vi "Extract Strings from Menu.vi"(8 "error in (no error)":errorcluster, 11 "Object in":refnum<class "Menu Data.lvclass">) -> (0 "error out":errorcluster, 3 "Object out":refnum<class "Menu Data.lvclass">)   [LabVIEW 2013, in "SET Project Data.lvlib" / "Menu Data.lvclass"]
uses:
  Menu Data.lvclass
  Menu Data.lvclass/Menu Data.ctl
  <vilib>/Utility/miscctls.llb/LVMenuShortCut.ctl
  Resource Data Class/Resource Data.lvclass
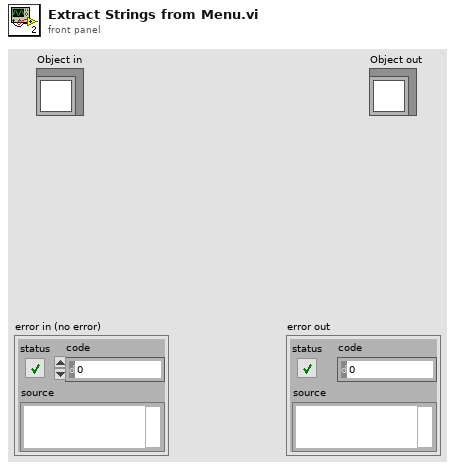
[diagram p1: front panel]
types:
  T1 = enum32{"Invalid", "Standard", "Closed", "Hidden", "Minimized", "Maximized"}
  T2 = typedef "LVMenuShortCut.ctl" = cluster{"Include Shift Key?":bool, "Include Ctrl Key?":bool, "Shortcut Key":string}
  T3 = cluster{"tag":string, "name":string, "short cut":T2, "enabled":bool, "checked":bool}[]
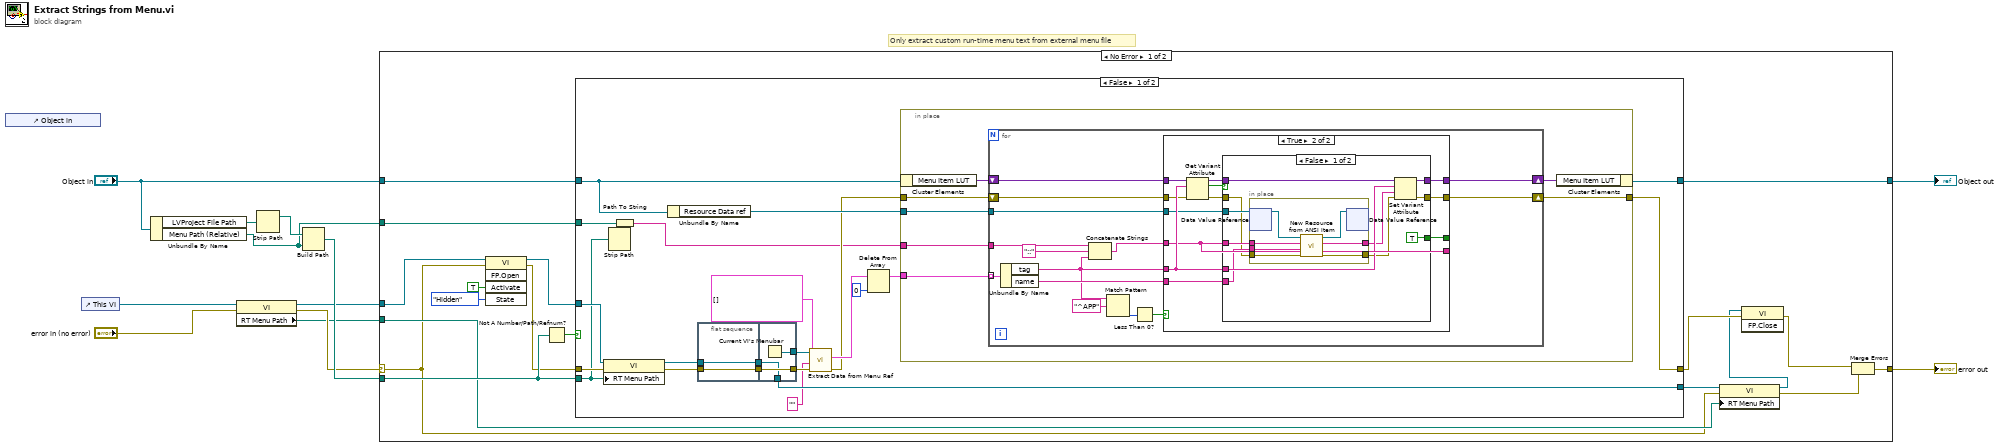
[diagram p0: block diagram]
diagram:
  # "Only extract custom run-time menu text from external menu file"
  n1 = control-ref of="Object in"() -> ()  [unwired: 1 out]
  n2 = control-ref of="This VI"() -> (w6:refnum<vi>)
  n3 = Unbundle By Name("Object in") -> ("LVProject File Path"=w11:path, "Menu Path (Relative)"=w1:path)
  n4 = property class="VI"(reference=w6, error in="error in (no error)") -> (reference out=w5:refnum<vi>, error out=w3:errorcluster, "RT Menu Path"=w2:path)
  n5 = Strip Path(path=w11) -> (stripped path=w12:path)  [unwired: 1 out]
  n6 = Build Path(base path=w12, name or relative path=w1) -> (appended path=w8:path)
  n7 = case shown="No Error" w3 {
    selector: w3 -> [w19 w118]
    tunnel: w5 -> [w23 _]
    tunnel: [w26 w118] -> w7
    tunnel: w8 -> [w29 _]
    tunnel: "Object in" -> [w28 w117]
    tunnel: [w27 w117] -> w9
    tunnel: w2 -> [w24 _]
    tunnel: w1 -> [w13 _]
    frame No Error {
      n8 = invoke class="VI" method="FP.Open"(reference=w23, error in=w19, "Activate"=TRUE ("Activate?"), "State"=T1."Hidden") -> (reference out=w22:refnum<vi>, error out=w18:errorcluster)  [unwired: 1 in, 3 out]
      n9 = Not A Number/Path/Refnum?(number/path/refnum=w29) -> (NaN/Path/Refnum?=w30:bool)
      n10 = case shown="False" w30 {
        tunnel: w22 -> [w51 w114]
        tunnel: w18 -> [w50 w116]
        tunnel: [w40 w116] -> w16
        tunnel: w29 -> [w44 _]
        tunnel: w28 -> [w43 w115]
        tunnel: [w45 w115] -> w27
        tunnel: [w36 w114] -> w17
        tunnel: w13 -> [w32 _]
        frame False {
          n11 = property class="VI"(reference=w51, error in=w50, "RT Menu Path"=w44) -> (reference out=w37:refnum<vi>, error out=w39:errorcluster)
          n12 = Strip Path(path=w44) -> ()  [unwired: 2 out]
          n13 = Path To String(path=w32) -> (string=w31:string)
          n14 = Unbundle By Name(w43) -> ("Resource Data ref"=w42:refnum<data-value>)
          n15 = flat-sequence {
            tunnel: w39 -> [w110]
            tunnel: [w110] -> w38
            tunnel: w37 -> [w109]
            tunnel: [w109] -> w35
            tunnel: [w113] -> w52
            tunnel: [w112] -> w49
            tunnel: w38 -> [w112]
            tunnel: [w111] -> w36
            tunnel: w35 -> [w111]
            frame #0 {
            }
            frame #1 {
              n16 = Current VI's Menubar() -> (w113:refnum<k9>)
            }
          }
          n17 = call "Extract Data from Menu Ref.vi"("error in (no error)"=w49, "Starting Tag"="", "Menu Items in"=T3 [], "menu reference"=w52) -> ("error out"=w41:errorcluster, "Menu Items out"=w48:T3)  [unwired: 5 in, 1 out]
          n18 = Delete From Array(array=w48, index=0) -> (array with subset deleted=w47:T3)  [unwired: 1 in, 1 out]
          n19 = in-place {
            in-place-border: w47 -> [w59]
            in-place-border: w31 -> [w56]
            in-place-border: w42 -> [w55]
            in-place-border: w41 -> [w54]
            in-place-border: [w53] -> w40
            n20 = in-place-cluster #1(w43) -> ("Menu Item LUT"=w58:variant)
            n21 = for {
              tunnel: w59 -> [w70] mode=indexing
              shift-right: [w67] -> w57
              shift-left: w58 -> [w68]
              tunnel: w56 -> [w66]
              tunnel: w55 -> [w63]
              shift-right: [w60] -> w53
              shift-left: w54 -> [w61]
              n22 = Unbundle By Name(w70) -> ("tag"=w64:string, "name"=w69:string)
              n23 = Concatenate Strings(w66, "::" ("string"), w64) -> (w62:string)
              n24 = Match Pattern(string=w64, regular expression="^APP") -> (offset past match=w72:i32)  [unwired: 1 in, 3 out]
              n25 = Less Than 0?(x=w72) -> (x < 0?=w71:bool)
              n26 = case shown="True" w71 {
                tunnel: w64 -> [_ w84]
                tunnel: w69 -> [_ w87]
                tunnel: w68 -> [w76 w86]
                tunnel: [w76 w88] -> w67
                tunnel: w63 -> [_ w82]
                tunnel: w62 -> [w74 w78]
                tunnel: w61 -> [w75 w80]
                tunnel: [w75 w79] -> w60
                tunnel: [w74 w78] -> _
                tunnel: [_ w77] -> _
                frame False {
                }
                frame True {
                  n27 = Get Variant Attribute(Variant=w86, name=w84, error in=w80) -> (duplicate Variant=w85:variant, found=w83:bool, error out=w81:errorcluster)  [unwired: 1 in, 1 out]
                  n28 = case shown="False" w83 {
                    tunnel: [w99 w108] -> w88
                    tunnel: w87 -> [w94 _]
                    tunnel: w85 -> [w98 w108]
                    tunnel: w84 -> [w97 _]
                    tunnel: w82 -> [w96 _]
                    tunnel: w78 -> [w95 _]
                    tunnel: w81 -> [w93 w107]
                    tunnel: [w90 w107] -> w79
                    tunnel: [TRUE _] -> w77
                    frame False {
                      n29 = in-place {
                        in-place-border: [w106] -> w91
                        in-place-border: [w105] -> w92
                        in-place-border: w95 -> [w104]
                        in-place-border: w93 -> [w103]
                        in-place-border: w94 -> [w102]
                        n30 = in-place-dvr #2(w96) -> (w101:refnum<class "Resource Data.lvclass">)  [unwired: 1 out]
                        n31 = call "New Resource from ANSI Item.vi"("error in (no error)"=w103, "Default String (ANSI)"=w102, "Tag (ANSI)"=w104, "LangFile in"=w101) -> ("error out"=w105:errorcluster, "RID"=w106:string, "LangFile out"=w100:refnum<class "Resource Data.lvclass">)  [unwired: 5 in]
                        n32 = in-place-dvr #2(w100) -> ()  [unwired: 2 out]
                      }
                      n33 = Set Variant Attribute(Variant=w98, name=w97, value=w91, error in=w92) -> (Variant out=w99:variant, error out=w90:errorcluster)  [unwired: 1 out]
                    }
                    frame True {
                      # "#TODO - Handle menu item update case"
                    }
                  }
                }
              }
            }
            n34 = in-place-cluster #1("Menu Item LUT"=w57) -> (w45:refnum<class "Menu Data.lvclass">)
          }
        }
        frame True {
        }
      }
      n35 = property class="VI"(reference=w17, error in=w19, "RT Menu Path"=w24) -> (reference out=w14:refnum<vi>, error out=w25:errorcluster)
      n36 = invoke class="VI" method="FP.Close"(reference=w14, error in=w16) -> (error out=w15:errorcluster)  [unwired: 1 in, 2 out]
      n37 = Merge Errors(w15, w25) -> (w26:errorcluster)
    }
    frame Error {
    }
  }
  "error out" <- w7
  "Object out" <- w9
